vi "Phasor Calibration v3.vi"(6 "Compute Lifetimes? (F)":bool, 8 "Error In":errorcluster, 9 "Phasor Frequency":dbl[unit], 10 "Calibration Phasor":T2, 11 "Measured Phasor":T1) -> (0 "Error Out":errorcluster, 1 "Calibrated Phase Lifetime":dbl[unit], 2 "IRF Calibrated Phasor":T1, 3 "Calibrated Phasor":T1, 4 "Calibrated Modulus Lifetime":dbl[unit], 5 "Calibrated?":bool)   [LabVIEW 2021, in "Phasor.lvlib"]
uses:
  Phasor.lvlib
  Phasor (g, s).ctl
  Calibration Phasor (m, phi).ctl
  7982dff7-fac1-446e-9812-be874fd64d1b.vi
  3b3d077d-b05d-4ac6-b92c-26b13ba21f37.vi
  b92aa7b5-96fb-4dd5-b5f8-7c0b6f61aa30.vi
  b92aa7b5-96fb-4dd5-b5f8-7c0b6f61aa30.vi/8a80743f-1319-44c8-96b0-3ef8fc688731.vi
  b92aa7b5-96fb-4dd5-b5f8-7c0b6f61aa30.vi/931f4f8f-d8c6-4056-833f-5c8fe97b24b9.vi
  <vilib>/Utility/error.llb/Error Cluster From Error Code.vi
  <vilib>/ErrorRing/Error Ring.xnode
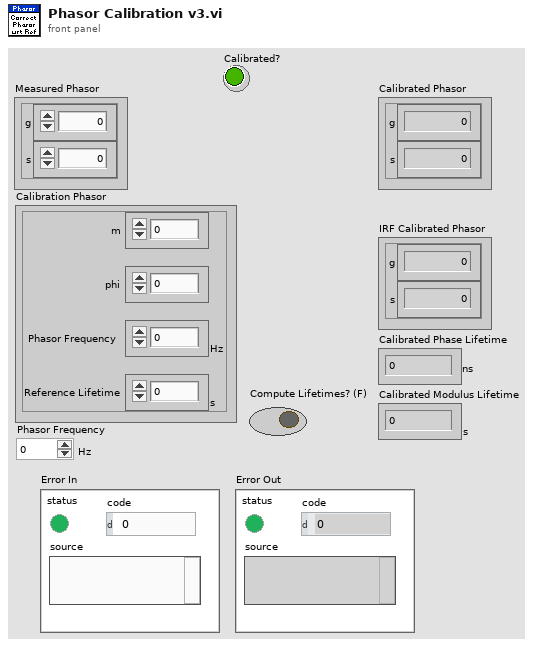
[diagram p1: front panel]
types:
  T1 = typedef "Phasor.lvlib/Phasor (g, s).ctl" = cluster{"g":dbl, "s":dbl}
  T2 = typedef "Phasor.lvlib/Calibration Phasor (m, phi).ctl" = cluster{"m":dbl, "phi":dbl, "Phasor Frequency":dbl[unit], "Reference Lifetime":dbl[unit]}
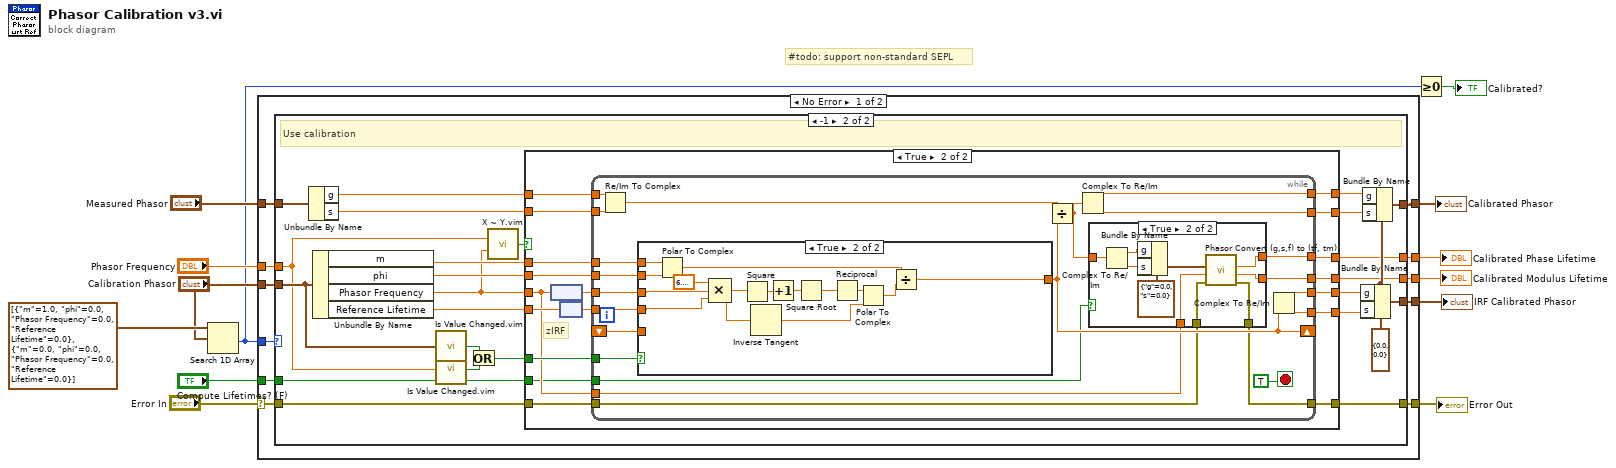
[diagram p0: block diagram]
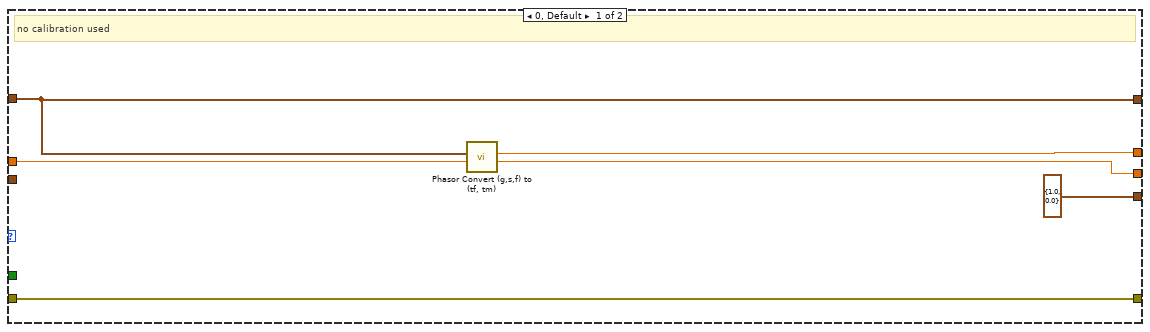
[diagram p2: hidden frame]
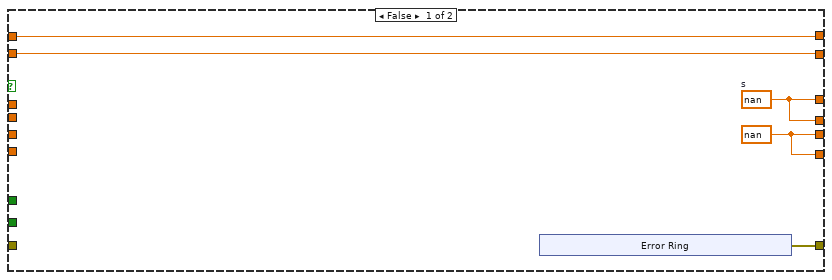
[diagram p3: hidden frame]
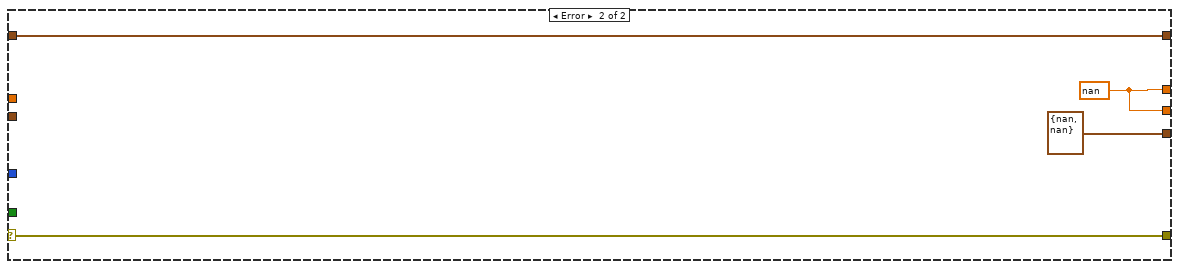
[diagram p6: hidden frame]
diagram:
  # "#todo: support non-standard SEPL"
  n1 = Search 1D Array(1D array=T2[] [{"m"=1.0, "phi"=0.0, "Phasor Frequency"=0.0, "Reference Lifetime"=0.0}, {"m"=0.0, "phi"=0.0, "Phasor Frequency"=0.0, "Reference Lifetime"=0.0}] ("Calibration Phasor"), element="Calibration Phasor") -> (index of element=w1:i32)  [unwired: 1 in]
  n2 = case shown="No Error" "Error In" {
    selector: "Error In" -> [w16 w132]
    tunnel: "Measured Phasor" -> [w24 w134]
    tunnel: [w23 w134] -> w12
    tunnel: [w22 T1 {"g"=nan, "s"=nan} ("Corrected Phasor")] -> w11
    tunnel: [w21 w131] -> w10
    tunnel: "Calibration Phasor" -> [w20 _]
    tunnel: w1 -> [w19 _]
    tunnel: "Compute Lifetimes? (F)" -> [w14 _]
    tunnel: "Phasor Frequency" -> [w18 _]
    tunnel: [w17 w132] -> w5
    tunnel: [w15 w131] -> w4
    frame No Error {
      n3 = case shown="-1" w19 {
        tunnel: w24 -> [w29 w55]
        tunnel: [w29 w47] -> w23
        tunnel: [T1 {"g"=1.0, "s"=0.0} ("Corrected Phasor") w46] -> w22
        tunnel: [w28 w42] -> w21
        tunnel: w20 -> [_ w36]
        tunnel: w18 -> [w27 w35]
        tunnel: [w26 w39] -> w17
        tunnel: w16 -> [w26 w38]
        tunnel: [w25 w37] -> w15
        tunnel: w14 -> [_ w31]
        frame 0, Default {
          # "no calibration used"
          n4 = call "Phasor Convert (g,s,f) to (tf, tm).vi"("Phasor Harmonic Frequency"=w27, "Phasor (g, s)"=w29) -> ("Modulus Lifetime"=w25:dbl[unit], "Phase Lifetime"=w28:dbl[unit])  [unwired: 7 in, 1 out]
        }
        frame -1 {
          w45 = T1 {"g"=0.0, "s"=0.0} ("Corrected Phasor")
          # "Use calibration"
          n5 = Unbundle By Name(w55) -> ("g"=w54:dbl, "s"=w53:dbl)
          n6 = Unbundle By Name(w36) -> ("m"=w52:dbl, "phi"=w51:dbl, "Phasor Frequency"=w41:dbl[unit], "Reference Lifetime"=w50:dbl[unit])
          n7 = call "Is Value Changed.vim"("value"=w36) -> ("changed or first call?"=w34:bool)
          n8 = call "Is Value Changed.vim"("value"=w35) -> ("changed or first call?"=w33:bool)
          n9 = Or(x=w34, y=w33) -> (x .or. y?=w32:bool)
          n10 = call "X ~ Y.vim"("X"=w35, "Y"=w41) -> ("X ~= Y?"=w40:bool)  [unwired: 13 in]
          n11 = case shown="True" w40 {
            tunnel: w54 -> [w60 w82]
            tunnel: w53 -> [w59 w81]
            tunnel: w52 -> [_ w80]
            tunnel: w51 -> [_ w79]
            tunnel: w50 -> [_ w77]
            tunnel: [w60 w75] -> w49
            tunnel: [w59 w74] -> w48
            tunnel: [w58 w73] -> w44
            tunnel: [w58 w72] -> w43
            tunnel: [w56 w71] -> w42
            tunnel: w32 -> [_ w70]
            tunnel: w41 -> [_ w67]
            tunnel: [w57 w66] -> w39
            tunnel: w38 -> [_ w68]
            tunnel: [w56 w69] -> w37
            tunnel: w31 -> [_ w65]
            frame False {
              w58 = nan
              w56 = dbl[unit] nan  # s
              n12 = xnode "Error Ring"() -> ("error out"=w57:errorcluster)
            }
            frame True {
              # "zIRF"
              n13 = node(w67) -> (w78:dbl)
              n14 = node(w77) -> (w76:dbl)
              n15 = while {
                tunnel: w70 -> [w103]
                tunnel: w80 -> [w102]
                tunnel: w79 -> [w101]
                tunnel: w78 -> [w96]
                tunnel: w76 -> [w100]
                tunnel: w81 -> [w98]
                tunnel: w82 -> [w99]
                tunnel: [w94] -> w75
                tunnel: [w95] -> w74
                tunnel: [w97] -> w71
                shift-right: [w90] -> _
                shift-left: _ -> [w93]
                tunnel: [w89] -> w73
                tunnel: [w88] -> w72
                tunnel: [w87] -> w69
                tunnel: w68 -> [w85]
                tunnel: w67 -> [w86]
                tunnel: [w84] -> w66
                tunnel: w65 -> [w83]
                stop <- TRUE stop-if-true
                n16 = Re/Im To Complex(1:w98, 2:w99) -> (0:w92:cdb)
                n17 = case shown="True" w103 {
                  tunnel: w102 -> [_ w130]
                  tunnel: w101 -> [_ w129]
                  tunnel: w96 -> [_ w128]
                  tunnel: w100 -> [_ w127]
                  tunnel: w93 -> [w116 _]
                  tunnel: [w116 w126] -> w90
                  frame False {
                  }
                  frame True {
                    n18 = Polar To Complex(1:w129, 2:w130) -> (0:w118:cdb)
                    n19 = Compound Arithmetic op=MULTIPLY(6.283185307179586, w128, w127) -> (w119:dbl)
                    n20 = Square(x=w119) -> (x^2=w124:dbl)
                    n21 = Inverse Tangent(1:w119) -> (0:w122:dbl)
                    n22 = Increment(x=w124) -> (x+1=w123:dbl)
                    n23 = Square Root(x=w123) -> (sqrt(x)=w120:dbl)
                    n24 = Reciprocal(x=w120) -> (1/x=w121:dbl)
                    n25 = Polar To Complex(1:w122, 2:w121) -> (0:w117:cdb)
                    n26 = Divide(x=w118, y=w117) -> (x/y=w126:cdb)
                  }
                }
                n27 = Divide(x=w92, y=w90) -> (x/y=w91:cdb)
                n28 = Complex To Re/Im(x + iy=w91) -> (x=w94:dbl, y=w95:dbl)
                n29 = case shown="True" w83 {
                  tunnel: [_ w115] -> w97
                  tunnel: w91 -> [_ w114]
                  tunnel: [_ w113] -> w87
                  tunnel: w86 -> [_ w112]
                  tunnel: w85 -> [w105 w111]
                  tunnel: [w105 w110] -> w84
                  frame False {
                  }
                  frame True {
                    n30 = Complex To Re/Im(x + iy=w114) -> (x=w108:dbl, y=w107:dbl)
                    n31 = Bundle By Name(cluster=T1 {"g"=0.0, "s"=0.0} ("Corrected Phasor"), "g"=w108, "s"=w107) -> (w106:T1)
                    n32 = call "Phasor Convert (g,s,f) to (tf, tm).vi"("Error In"=w111, "Phasor Harmonic Frequency"=w112, "Phasor (g, s)"=w106) -> ("Error Out"=w110:errorcluster, "Modulus Lifetime"=w113:dbl[unit], "Phase Lifetime"=w115:dbl[unit])  [unwired: 6 in]
                  }
                }
                n33 = Complex To Re/Im(x + iy=w90) -> (x=w89:dbl, y=w88:dbl)
              }
            }
          }
          n34 = Bundle By Name(cluster=w45, "g"=w44, "s"=w43) -> (w46:T1)
          n35 = Bundle By Name(cluster=w45, "g"=w49, "s"=w48) -> (w47:T1)
        }
      }
    }
    frame Error {
      w131 = dbl[unit] nan ("Phase Lifetime")
    }
  }
  "Calibrated Phasor" <- w12
  "IRF Calibrated Phasor" <- w11
  "Calibrated Phase Lifetime" <- w10
  "Error Out" <- w5
  "Calibrated Modulus Lifetime" <- w4
  n36 = Greater Or Equal To 0?(x=w1) -> (x >= 0?=→"Calibrated?":bool)
